vi "tab init.vi"() -> (3 "appended array":string[][](array[string]))   [LabVIEW 2019]
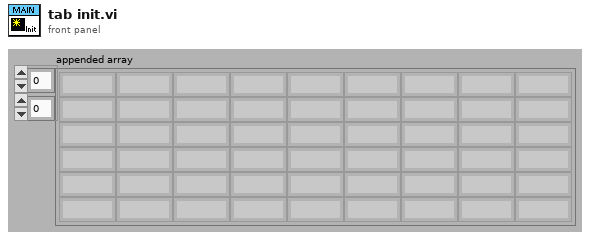
[diagram p1: front panel]
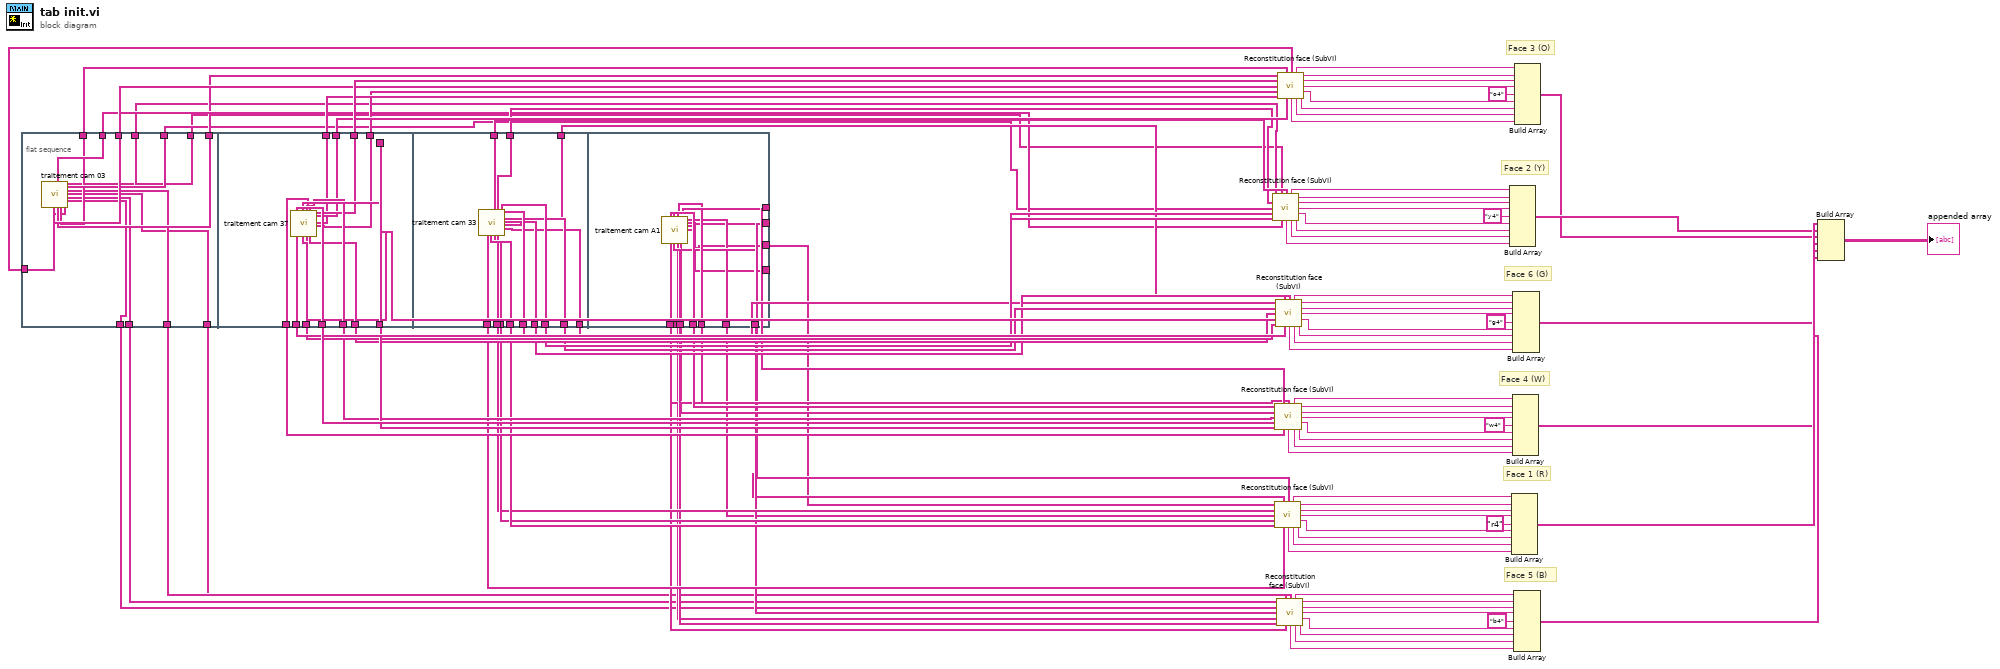
[diagram p0: block diagram]
diagram:
  # "Face 6 (G)"
  # "Face 5 (B)"
  # "Face 4 (W)"
  # "Face 3 (O)"
  # "Face 2 (Y)"
  # "Face 1 (R)"
  n1 = flat-sequence {
    tunnel: [w121] -> w12
    tunnel: [w120] -> w11
    tunnel: [w119] -> w10
    tunnel: [w118] -> w9
    tunnel: [w117] -> w8
    tunnel: [w116] -> w7
    tunnel: [w115] -> w6
    tunnel: [w114] -> w5
    tunnel: [w113] -> w4
    tunnel: [w112] -> w3
    tunnel: [w111] -> w2
    tunnel: [w110] -> w1
    tunnel: [w133] -> w48
    tunnel: [w132] -> w47
    tunnel: [w131] -> w46
    tunnel: [w130] -> w45
    tunnel: [w129] -> w44
    tunnel: [w122] -> w43
    tunnel: [w128] -> w42
    tunnel: [w127] -> w41
    tunnel: [w126] -> w40
    tunnel: [w125] -> w39
    tunnel: [w124] -> w38
    tunnel: [w123] -> w37
    tunnel: [w145] -> w36
    tunnel: [w144] -> w35
    tunnel: [w143] -> w34
    tunnel: [w142] -> w33
    tunnel: [w141] -> w32
    tunnel: [w140] -> w31
    tunnel: [w139] -> w30
    tunnel: [w138] -> w29
    tunnel: [w137] -> w28
    tunnel: [w136] -> w27
    tunnel: [w135] -> w26
    tunnel: [w134] -> w25
    tunnel: [w157] -> w24
    tunnel: [w156] -> w23
    tunnel: [w155] -> w22
    tunnel: [w154] -> w21
    tunnel: [w153] -> w20
    tunnel: [w152] -> w19
    tunnel: [w151] -> w18
    tunnel: [w150] -> w17
    tunnel: [w149] -> w16
    tunnel: [w148] -> w15
    tunnel: [w147] -> w14
    tunnel: [w146] -> w13
    frame #0 {
      n2 = call "traitement cam 03.vi"() -> ("Couleur carré 12 (3,6)"=w121:string[], "Couleur carré 4 (2,9)"=w120:string[], "Couleur carré 9 (3,3)"=w119:string[], "Couleur carré 3 (2,6)"=w118:string[], "Couleur carré 10 (3,2)"=w117:string[], "Couleur carré 2 (2,3)"=w116:string[], "Couleur carré 11 (3,1)"=w110:string[], "Couleur carré 1 (2,2)"=w115:string[], "Couleur carré 6 (5,1)"=w114:string[], "Couleur carré 7 (5,2)"=w113:string[], "Couleur carré 8 (5,3)"=w112:string[], "Couleur carré 5 (5,4)"=w111:string[])  [unwired: 15 in, 1 out]
    }
    frame #1 {
      n3 = call "traitement cam 37.vi"() -> ("Couleur carré 8 (4,7)"=w133:string[], "Couleur carré 11 (6,9)"=w132:string[], "Couleur carré 7 (4,8)"=w131:string[], "Couleur carré 10 (6,8)"=w130:string[], "Couleur carré 6 (4,9)"=w129:string[], "Couleur carré 9 (6,7)"=w122:string[], "Couleur carré 5 (4,6)"=w128:string[], "Couleur carré 12 (6,6)"=w127:string[], "Couleur carré 1 (3,4)"=w126:string[], "Couleur carré 2 (3,9)"=w125:string[], "Couleur carré 3 (3,8)"=w124:string[], "Couleur carré 4 (3,7)"=w123:string[])  [unwired: 15 in, 1 out]
    }
    frame #2 {
      n4 = call "traitement cam 33.vi"() -> ("Couleur carré 11 (1,9)"=w145:string[], "Couleur carré 10  (1,8)"=w144:string[], "Couleur carré 4 (2,1)"=w143:string[], "Couleur carré 9 (1,7)"=w142:string[], "Couleur carré 3 (2,4)"=w141:string[], "Couleur carré 12 (1,4)"=w140:string[], "Couleur carré 2 (2,7)"=w139:string[], "Couleur carré 1 (2,8)"=w138:string[], "Couleur carré 5 (6,4)"=w137:string[], "Couleur carré 6 (6,1)"=w136:string[], "Couleur carré 7 (6,2)"=w135:string[], "Couleur carré 8 (6,3)"=w134:string[])  [unwired: 15 in, 1 out]
    }
    frame #3 {
      n5 = call "traitement cam A1.vi"() -> ("Couleur carré 8 (4,3)"=w157:string[], "Couleur carré 11 (5,9)"=w156:string[], "Couleur carré 7 (4,2)"=w155:string[], "Couleur carré 10 (5,8)"=w154:string[], "Couleur carré 6 (4,1)"=w153:string[], "Couleur carré 9 (5,7)"=w152:string[], "Couleur carré 5 (4,4)"=w151:string[], "Couleur carré 12 (5,6)"=w150:string[], "Couleur carré 1 (1,6)"=w149:string[], "Couleur carré 2 (1,1)"=w148:string[], "Couleur carré 3 (1,2)"=w147:string[], "Couleur carré 4 (1,3)"=w146:string[])  [unwired: 15 in, 1 out]
    }
  }
  n6 = call "Reconstitution face (SubVI).vi"("Couleur carrée  2"=w7, "Couleur carrée  1"=w6, "Couleur carrée 0"=w34, "Couleur carrée  3"=w32, "Couleur carrée  5"=w9, "Couleur carrée  6"=w30, "Couleur carrée  7"=w29, "Couleur carrée  8"=w11) -> ("Couleur 0"=w92:string, "Couleur 1"=w93:string, "Couleur  2"=w94:string, "Couleur 3"=w95:string, "Couleur 5"=w96:string, "Couleur 8"=w98:string, "Couleur 7"=w99:string, "Couleur 6"=w97:string)
  n7 = call "Reconstitution face (SubVI).vi"("Couleur carrée  2"=w13, "Couleur carrée  1"=w14, "Couleur carrée 0"=w15, "Couleur carrée  3"=w31, "Couleur carrée  5"=w16, "Couleur carrée  6"=w33, "Couleur carrée  7"=w35, "Couleur carrée  8"=w36) -> ("Couleur 0"=w109:string, "Couleur 1"=w108:string, "Couleur  2"=w107:string, "Couleur 3"=w106:string, "Couleur 5"=w105:string, "Couleur 8"=w103:string, "Couleur 7"=w102:string, "Couleur 6"=w104:string)
  n8 = call "Reconstitution face (SubVI).vi"("Couleur carrée  2"=w24, "Couleur carrée  1"=w22, "Couleur carrée 0"=w20, "Couleur carrée  3"=w18, "Couleur carrée  5"=w42, "Couleur carrée  6"=w48, "Couleur carrée  7"=w46, "Couleur carrée  8"=w44) -> ("Couleur 0"=w74:string, "Couleur 1"=w75:string, "Couleur  2"=w76:string, "Couleur 3"=w77:string, "Couleur 5"=w78:string, "Couleur 8"=w80:string, "Couleur 7"=w81:string, "Couleur 6"=w79:string)
  n9 = call "Reconstitution face (SubVI).vi"("Couleur carrée  2"=w25, "Couleur carrée  1"=w26, "Couleur carrée 0"=w27, "Couleur carrée  3"=w28, "Couleur carrée  5"=w41, "Couleur carrée  6"=w43, "Couleur carrée  7"=w45, "Couleur carrée  8"=w47) -> ("Couleur 0"=w56:string, "Couleur 1"=w57:string, "Couleur  2"=w58:string, "Couleur 3"=w59:string, "Couleur 5"=w60:string, "Couleur 8"=w62:string, "Couleur 7"=w63:string, "Couleur 6"=w61:string)
  n10 = call "Reconstitution face (SubVI).vi"("Couleur carrée  2"=w3, "Couleur carrée  1"=w4, "Couleur carrée 0"=w5, "Couleur carrée  3"=w2, "Couleur carrée  5"=w17, "Couleur carrée  6"=w19, "Couleur carrée  7"=w21, "Couleur carrée  8"=w23) -> ("Couleur 0"=w73:string, "Couleur 1"=w72:string, "Couleur  2"=w71:string, "Couleur 3"=w70:string, "Couleur 5"=w69:string, "Couleur 8"=w67:string, "Couleur 7"=w66:string, "Couleur 6"=w68:string)
  n11 = call "Reconstitution face (SubVI).vi"("Couleur carrée  2"=w10, "Couleur carrée  1"=w8, "Couleur carrée 0"=w1, "Couleur carrée  3"=w40, "Couleur carrée  5"=w12, "Couleur carrée  6"=w37, "Couleur carrée  7"=w38, "Couleur carrée  8"=w39) -> ("Couleur 0"=w91:string, "Couleur 1"=w90:string, "Couleur  2"=w89:string, "Couleur 3"=w88:string, "Couleur 5"=w87:string, "Couleur 8"=w85:string, "Couleur 7"=w84:string, "Couleur 6"=w86:string)
  n12 = Build Array(w92, w93, w94, w95, "y4" ("element"), w96, w97, w99, w98) -> (w54:string[])
  n13 = Build Array(w109, w108, w107, w106, "r4" ("element"), w105, w104, w102, w103) -> (w55:string[])
  n14 = Build Array(w74, w75, w76, w77, "w4" ("element"), w78, w79, w81, w80) -> (w52:string[])
  n15 = Build Array(w56, w57, w58, w59, "g4" ("element"), w60, w61, w63, w62) -> (w50:string[])
  n16 = Build Array(w73, w72, w71, w70, "b4" ("element"), w69, w68, w66, w67) -> (w51:string[])
  n17 = Build Array(w91, w90, w89, w88, "o4" ("element"), w87, w86, w84, w85) -> (w53:string[])
  n18 = Build Array(w55, w54, w53, w52, w51, w50) -> (→"appended array":string[][])
